vi "19.2.-Data Socket de VIs con Código de LabVIEW (SLAVE).vi"() -> ()   [LabVIEW 2017]
panel:
  out "error out":errorcluster
  in  "Waveform Graph 2":dbl[](graph)
  out "Waveform Graph":dbl[](graph)
  in  "URL":string
  in  "stop":bool
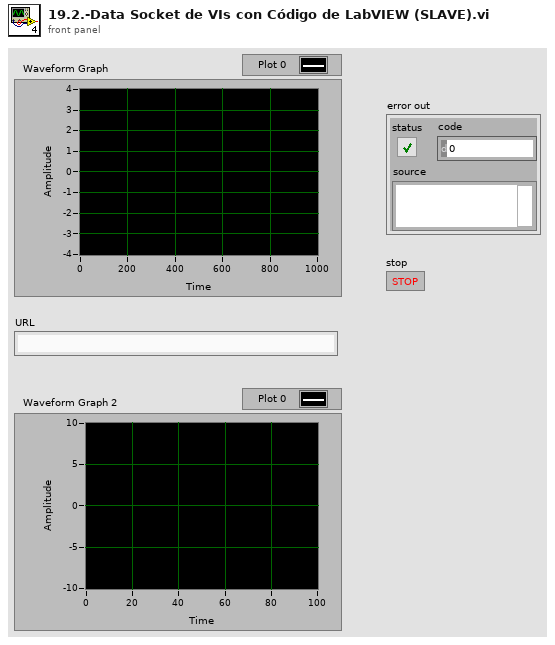
[diagram p1: front panel]
types:
  T1 = enum16{"Read", "Write", "ReadWrite", "BufferedRead", "BufferedReadWrite"}
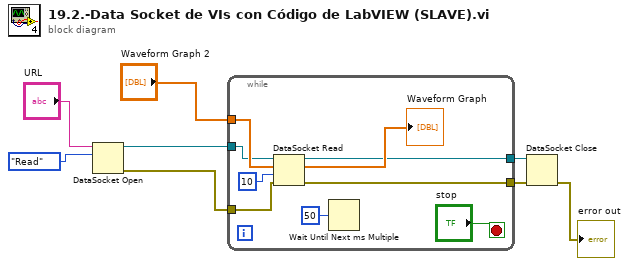
[diagram p0: block diagram]
diagram:
  n1 = DataSocket Open(10:T1."Read" ("mode"), 11:"URL") -> (0:w5:errorcluster, 3:w6:refnum<k13>)  [unwired: 2 in]
  n2 = while {
    tunnel: w6 -> [w11]
    tunnel: w5 -> [w15]
    tunnel: "Waveform Graph 2" -> [w13]
    tunnel: [w10] -> w3
    tunnel: [w9] -> w2
    stop <- "stop" stop-if-true
    n3 = DataSocket Read(8:w15, 9:10 ("ms timeout (10000)"), 10:w13, 11:w11) -> (0:w9:errorcluster, 2:→"Waveform Graph":dbl[], 3:w10:refnum<k13>)  [unwired: 1 in, 4 out]
    n4 = Wait Until Next ms Multiple(millisecond multiple=u32 50) -> ()  [unwired: 1 out]
  }
  n5 = DataSocket Close(8:w2, 11:w3) -> (0:→"error out":errorcluster)  [unwired: 1 in, 1 out]
